vi "ReadConfig.vi"(8 "error in (no error)":errorcluster, 11 "GRMActor in":refnum<class "DataLoggerUI.lvclass">) -> (0 "error out":errorcluster, 3 "GRMActor out":refnum<class "DataLoggerUI.lvclass">)   [LabVIEW 2020, in "DataLogger.lvlib" / "DataLoggerUI.lvlib" / "DataLoggerUI.lvclass"]
uses:
  DataLoggerUI.lvclass
  DataLoggerUI.lvclass/DataLoggerUI.ctl
  Hardware Abstraction Layer/Component/GenericActor/GenericActor/GenericController.lvclass
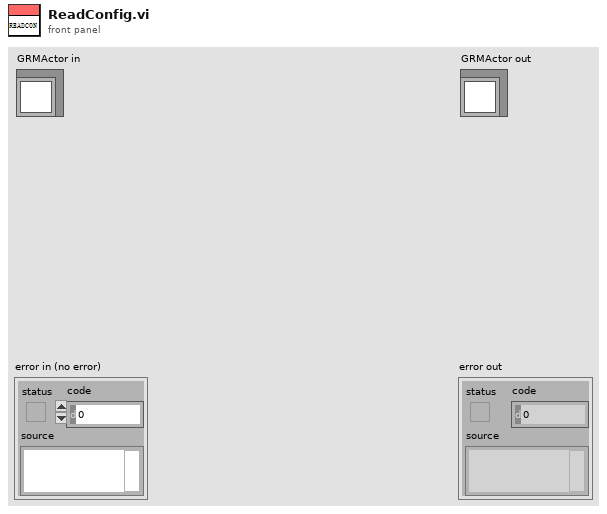
[diagram p1: front panel]
types:
  T1 = typedef "NI_LVConfig.lvlib/Config Data RefNum.ctl" = refnum<k1>
  T2 = cluster{"Values[0]":bool, "Values[1]":bool, "Values[2]":bool}
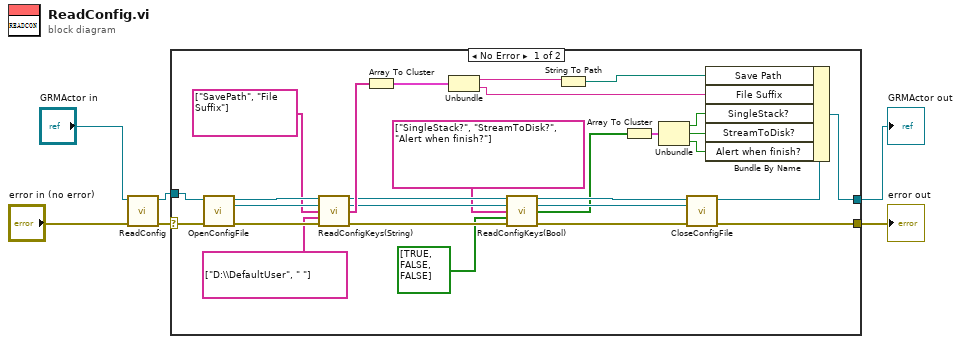
[diagram p0: block diagram]
diagram:
  n1 = call-parent "ReadConfig.vi"("error in (no error)"="error in (no error)", "GRMActor in"="GRMActor in") -> ("error out"=w4:errorcluster, "GRMActor out"=w3:refnum<class "DataLoggerUI.lvclass">)  [unwired: 8 in]
  n2 = case shown="No Error" w4 {
    selector: w4 -> [w34 w35]
    tunnel: [w27 w35] -> w1
    tunnel: [w29 w36] -> w2
    tunnel: w3 -> [w33 w36]
    frame No Error {
      n3 = call-dynamic "OpenConfigFile.vi"("error in (no error)"=w34, "GRMActor in"=w33) -> ("error out"=w32:errorcluster, "refnum"=w28:T1, "GRMActor out"=w30:refnum<class "DataLoggerUI.lvclass">)  [unwired: 7 in]
      n4 = call-dynamic "ReadConfigKeys(String).vi"("GRMActor in"=w30, "Config Refnum"=w28, "Keys"=string[] ["SavePath", "File Suffix"] ("Values"), "Values"=string[] ["D:\\DefaultUser", " "], "error in (no error)"=w32) -> ("GRMActor out"=w21:refnum<class "DataLoggerUI.lvclass">, "Config Refnum dup"=w19:T1, "Values"=w25:string[], "error out"=w31:errorcluster)  [unwired: 7 in]
      n5 = Array To Cluster(array=w25) -> (cluster=w10:cluster{"Values[0]":string, "Values[1]":string})
      n6 = Unbundle(w10) -> ("Values[0]"=w9:string, "Values[1]"=w8:string)
      n7 = call-dynamic "ReadConfigKeys(Bool).vi"("GRMActor in"=w21, "Config Refnum"=w19, "Keys"=string[] ["SingleStack?", "StreamToDisk?", "Alert when finish?"], "Values"=bool[] [TRUE, FALSE, FALSE], "error in (no error)"=w31) -> ("GRMActor out"=w20:refnum<class "DataLoggerUI.lvclass">, "Config Refnum dup"=w18:T1, "Values"=w15:bool[], "error out"=w22:errorcluster)  [unwired: 7 in]
      n8 = String To Path(string=w9) -> (path=w7:path)
      n9 = Array To Cluster(array=w15) -> (cluster=w14:T2)
      n10 = Unbundle(w14) -> ("Values[0]"=w13:bool, "Values[1]"=w12:bool, "Values[2]"=w11:bool)
      n11 = call-dynamic "CloseConfigFile.vi"("error in (no error)"=w22, "refnum"=w18, "GRMActor in"=w20) -> ("error out"=w27:errorcluster, "GRMActor out"=w26:refnum<class "DataLoggerUI.lvclass">)  [unwired: 7 in]
      n12 = Bundle By Name(cluster=w26, "Save Path"=w7, "File Suffix"=w8, "SingleStack?"=w13, "StreamToDisk?"=w12, "Alert when finish?"=w11) -> (w29:refnum<class "DataLoggerUI.lvclass">)
    }
    frame Error {
    }
  }
  "error out" <- w1
  "GRMActor out" <- w2
